vi "Measurement.Free.OnMeasured.vi"(8 "error in (no error)":errorcluster, 10 "Measured":T1, 11 "Measurement.Free":refnum<class "Measurement.Free.lvclass">) -> (0 "error out":errorcluster, 3 "Measurement.Free out":refnum<class "Measurement.Free.lvclass">)   [LabVIEW 2017, in "Measurement.Free.lvclass"]
doc: "---------------------------------------------------------------\nJKI State Machine Objects™\nhttp://jki.net/state-machine-objects/\nCopyright (C) 2005-2015, JKI <info@jki.net>\nALL RIGHTS RESERVEDJKI State Machine Objects (SMO) 1.0.0.4\nJKI - JKI\nCopyright (c) 2015, JKI"
uses:
  Measurement.Free.lvclass
  Typedefs/Measurement.Free.Measured.ctl
  Measurement.Free.lvclass/Measurement.Free.ctl
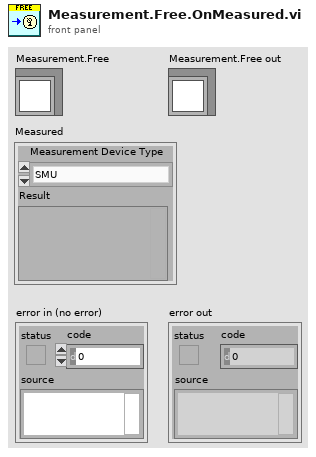
[diagram p1: front panel]
types:
  T1 = typedef "Measurement.Free.lvclass/Measurement.Free.Measured.ctl" = cluster{"Measurement Device Type":enum16{"SMU", "LIA", "OPM"}, "Result":variant}
  T2 = typedef "Measurement.Free.lvclass/PrivateData--Ref.ctl" = refnum<data-value>
  T3 = typedef "Measurement.Free.lvclass/PrivateData--Cluster.ctl" = cluster{"Configuration":T4, "Public Events":T14, "Private Events":T15}
  T4 = typedef "Measurement.Free.lvclass/Configuration--Cluster.ctl" = cluster{"Measurement.Type":enum16{"Free", "I/V Curve", "Wavelength sweeping", "Photocurrent mapping"}, "Hardware":T5}
  T5 = typedef "Measurement.Free.lvclass/Configuration.Hardware--Cluster.ctl" = cluster{"SMU":T6, "LIA":T8, "OPM":T10, "OPA":T12}
  T6 = typedef "Measurement.Free.lvclass/Configuration.SMU--Cluster.ctl" = cluster{"Enable":bool, "SMU Model":string, "Configuration":T7}
  T7 = typedef "SMU.lvclass/Configuration--Cluster.ctl" = cluster{"VISA Resource":string, "Channel":string}
  T8 = typedef "Measurement.Free.lvclass/Configuration.LIA--Cluster.ctl" = cluster{"Enable":bool, "LIA Model":string, "Configuration":T9}
  T9 = typedef "LIA.lvclass/Configuration--Cluster.ctl" = cluster{"VISA Resource":string}
  T10 = typedef "Measurement.Free.lvclass/Configuration.OPM--Cluster.ctl" = cluster{"Enable":bool, "OPM Model":string, "Configuration":T11}
  T11 = typedef "OPM.lvclass/Configuration--Cluster.ctl" = cluster{"VISA Resource":string}
  T12 = typedef "Measurement.Free.lvclass/Configuration.OPA--Cluster.ctl" = cluster{"Enable":bool, "OPA Model":string, "Configuration":T13}
  T13 = typedef "OPA.lvclass/Configuration--Cluster.ctl" = cluster{"Serial Number":string}
  T14 = typedef "Measurement.Free.lvclass/PublicEvents--Cluster.ctl" = cluster{"Initialized":refnum<user-event>, "Measured":refnum<user-event>}
  T15 = typedef "Measurement.Free.lvclass/PrivateEvents--Cluster.ctl" = cluster{"Initialize":refnum<user-event>}
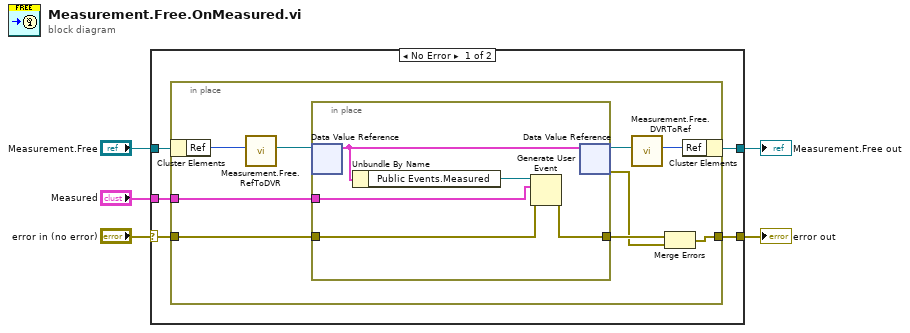
[diagram p0: block diagram]
diagram:
  n1 = case shown="No Error" "error in (no error)" {
    selector: "error in (no error)" -> [w8 w26]
    tunnel: [w7 w26] -> w4
    tunnel: [w9 w25] -> w5
    tunnel: "Measurement.Free" -> [w10 w25]
    tunnel: "Measured" -> [w6 _]
    frame No Error {
      n2 = in-place {
        in-place-border: w8 -> [w19]
        in-place-border: [w16] -> w7
        in-place-border: w6 -> [w11]
        n3 = in-place-cluster #1(w10) -> ("Ref"=w15:u32)
        n4 = call "Measurement.Free.RefToDVR.vi"("Ref"=w15) -> ("Ref"=w13:T2)  [unwired: 10 in]
        n5 = in-place {
          in-place-border: w19 -> [w22]
          in-place-border: [w21] -> w18
          in-place-border: w11 -> [w20]
          n6 = in-place-dvr #2(w13) -> (w24:T3)  [unwired: 1 out]
          n7 = Unbundle By Name(w24) -> ("Public Events.Measured"=w23:refnum<user-event>)
          n8 = Generate User Event(user event=w23, event data cluster=w20, error in=w22) -> (error out=w21:errorcluster)  [unwired: 1 in, 1 out]
          n9 = in-place-dvr #2(w24) -> (w14:T2, w17:errorcluster)
        }
        n10 = call "Measurement.Free.DVRToRef.vi"("Ref"=w14) -> ("Ref"=w12:u32)  [unwired: 10 in]
        n11 = Merge Errors(w18, w17) -> (w16:errorcluster)
        n12 = in-place-cluster #1("Ref"=w12) -> (w9:refnum<class "Measurement.Free.lvclass">)
      }
    }
    frame Error {
    }
  }
  "error out" <- w4
  "Measurement.Free out" <- w5
